vi "password.vi"() -> ()   [LabVIEW 2018]
panel:
  out "String 2":string
  in  "String":string
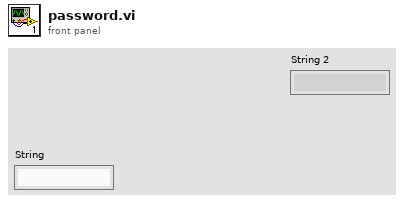
[diagram p1: front panel]
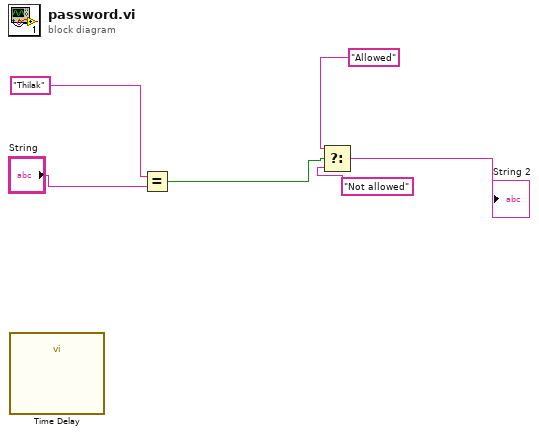
[diagram p0: block diagram]
diagram:
  n1 = call "Time Delay"() -> ()  [unwired: 11 in, 1 out]
  n2 = Equal?(x="Thilak", y="String") -> (x = y?=w4:bool)
  n3 = Select(t="Allowed", s=w4, f="Not allowed") -> (s? t:f=→"String 2":string)
